vi "XML to IO Channels.vi"(0 "XML Data":string) -> ()   [LabVIEW 2013]
uses:
  Types/IO Channels.ctl
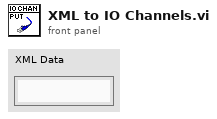
[diagram p1: front panel]
types:
  T1 = typedef "IO Channels.ctl" = cluster{"Division Input Channel":string, "Sum Input Channel":string, "X Input Channel":string, "X Output Channel":string, "Y Input Channel":string, "Y Output Channel":string, "Z Input Channel":string, "Z Output Channel":string, "Version":string}
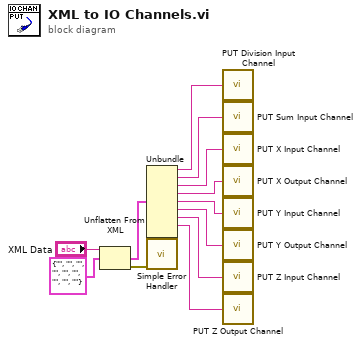
[diagram p0: block diagram]
diagram:
  n1 = Unflatten From XML(xml string="XML Data", type=T1 {"Division Input Channel"="", "Sum Input Channel"="", "X Input Channel"="", "X Output Channel"="", "Y Input Channel"="", "Y Output Channel"="", "Z Input Channel"="", "Z Output Channel"="", "Version"=""} ("IO Channels")) -> (value=w9:T1, error out=w12:errorcluster)  [unwired: 1 in]
  n2 = Unbundle(w9) -> ("Division Input Channel"=w4:string, "Sum Input Channel"=w5:string, "X Input Channel"=w6:string, "X Output Channel"=w8:string, "Y Input Channel"=w7:string, "Y Output Channel"=w3:string, "Z Input Channel"=w2:string, "Z Output Channel"=w1:string)  [unwired: 1 out]
  n3 = call <vilib>:"Simple Error Handler.vi"("error in (no error)"=w12) -> ()  [unwired: 4 in, 5 out]
  n4 = call "PUT Division Input Channel.vi"("Division Input Channel"=w4) -> ()
  n5 = call "PUT Sum Input Channel.vi"("Sum Input Channel"=w5) -> ()
  n6 = call "PUT X Input Channel.vi"("X Input Channel"=w6) -> ()
  n7 = call "PUT X Output Channel.vi"("X Output Channel"=w8) -> ()
  n8 = call "PUT Y Input Channel.vi"("Y Input Channel"=w7) -> ()
  n9 = call "PUT Y Output Channel.vi"("Y Output Channel"=w3) -> ()
  n10 = call "PUT Z Input Channel.vi"("Z Input Channel"=w2) -> ()
  n11 = call "PUT Z Output Channel.vi"("Z Output Channel"=w1) -> ()
